vi "Experiment header-Save_Load STATS section.vi"(4 "Logging queue element":T2={"Imaging Protocol"=enum."Live Imaging", "Number of Trials"=0, "Frame Size"=0, "# Averaged frames"=0, "Dwell time (us)"=0.1, "Index of Z-plane"=0, "Timelapse?"=FALSE, "Logging process is active"=FALSE, "Speed logging enabled"=FALSE, "tdms file ref"=refnum, "path"=path "", "Trial Number"=0, "Expected # points acquired"=FALSE, "Manually stopped"=FALSE, "Ch0 data"=[], "Ch1 data"=[], "Last trial"=FALSE, "Points acquired"={"Ch0 last trial"=0, "Ch1 last trial"=0, "All trials"=0}} {"Frame Size" items=["100X100"=100, "128X128"=128, "200X200"=200, "256X256"=256, "512X512"=512, "1024x1024"=1024, "2048x2048"=2048]; "Dwell time (us)" format="%#.6g"}, 8 "error in (no error)":errorcluster, 10 "Function":enum16{"Write", "Read"}(ring), 11 "Experiment folder path":path) -> (0 "error out":errorcluster, 1 "Read values":T1, 2 "Acquisition time unknown":bool)   [LabVIEW 2013]
uses:
  Typedefs/Logging queue element.ctl
  Typedefs/Imaging Protocols enum.ctl
  Typedefs/Frame Size.ctl
  Typedefs/Acquired points count.ctl
  Typedefs/Test header stats cluster.ctl
  <vilib>/Utility/config.llb/Read Key (Double).vi
  <vilib>/Utility/config.llb/Write Key (Double).vi
  Global Variables/General Globals.vi
  <vilib>/Utility/config.llb/NI_LVConfig.lvlib
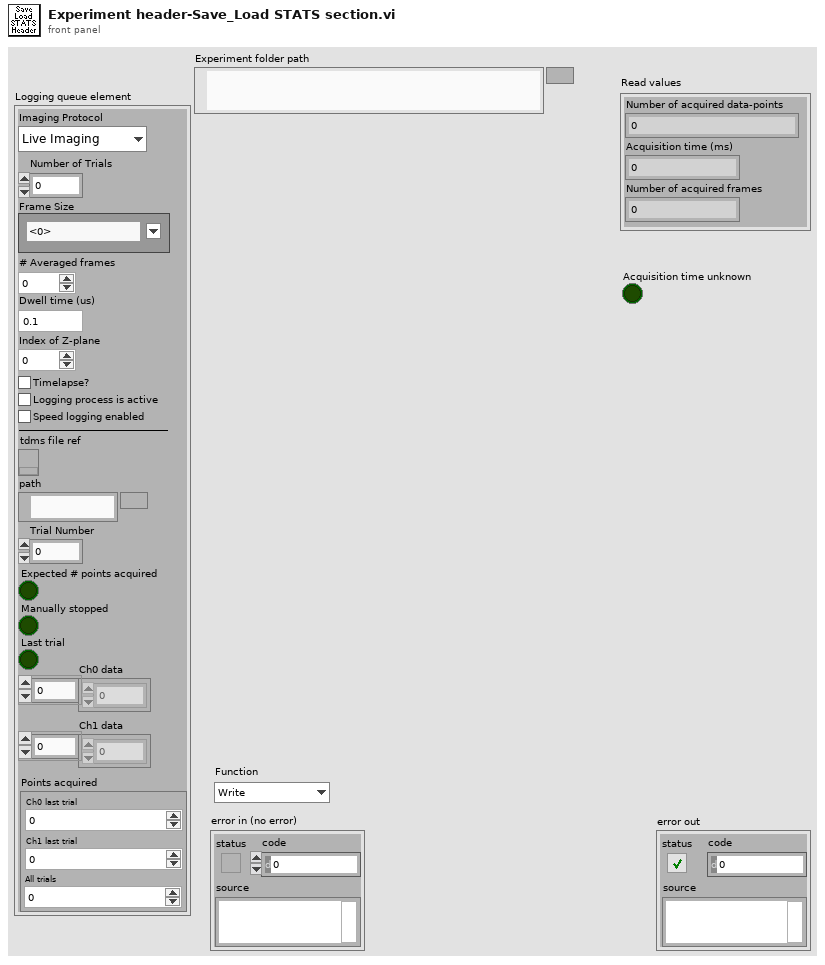
[diagram p1: front panel]
types:
  T1 = typedef "Test header stats cluster.ctl" = cluster{"Number of acquired data-points":dbl, "Acquisition time (ms)":dbl, "Number of acquired frames":dbl}
  T2 = typedef "Logging queue element.ctl" = cluster{"Imaging Protocol":T3, "Number of Trials":u16, "Frame Size":T4, "# Averaged frames":u16, "Dwell time (us)":dbl, "Index of Z-plane":i32, "Timelapse?":bool, "Logging process is active":bool, "Speed logging enabled":bool, "tdms file ref":refnum<k34>, "path":path, "Trial Number":i32, "Expected # points acquired":bool, "Manually stopped":bool, "Ch0 data":u32[], "Ch1 data":u32[], "Last trial":bool, "Points acquired":T5}
  T3 = typedef "Imaging Protocols enum.ctl" = enum16{"AOL Z-Stack", "Motor Z Stack", "Functional Acquisition", "Single Plane Acquisition", "Volume Acquisition", "Live Imaging", "Live Plane Imaging", "Live Volume Imaging"}
  T4 = typedef "Frame Size.ctl" = u16
  T5 = typedef "Acquired points count.ctl" = cluster{"Ch0 last trial":u64, "Ch1 last trial":u64, "All trials":u64}
  T6 = typedef "Fixed strings.ctl" = cluster{"ROI file name":string, "Normalised ROI file name":string, "Zplane Pockels values file name":string, "Functional data folder name":string, "Experiment Header file name":string, "Z-stack images folder name":string, "Groups setup rel. path":string, "Groups text file rel. path":string, "TDMS files folder name (F.img)":string, "TDMS files folder name (V.acq)":string, "TDMS files folder name (Pl.acq)":string, "Cycle rel times sequence file":string, "Dynamically called VIs folder name":string, "Time Series folder base name":string}
  T7 = typedef "NI_LVConfig.lvlib/Config Data RefNum.ctl" = refnum<k1>
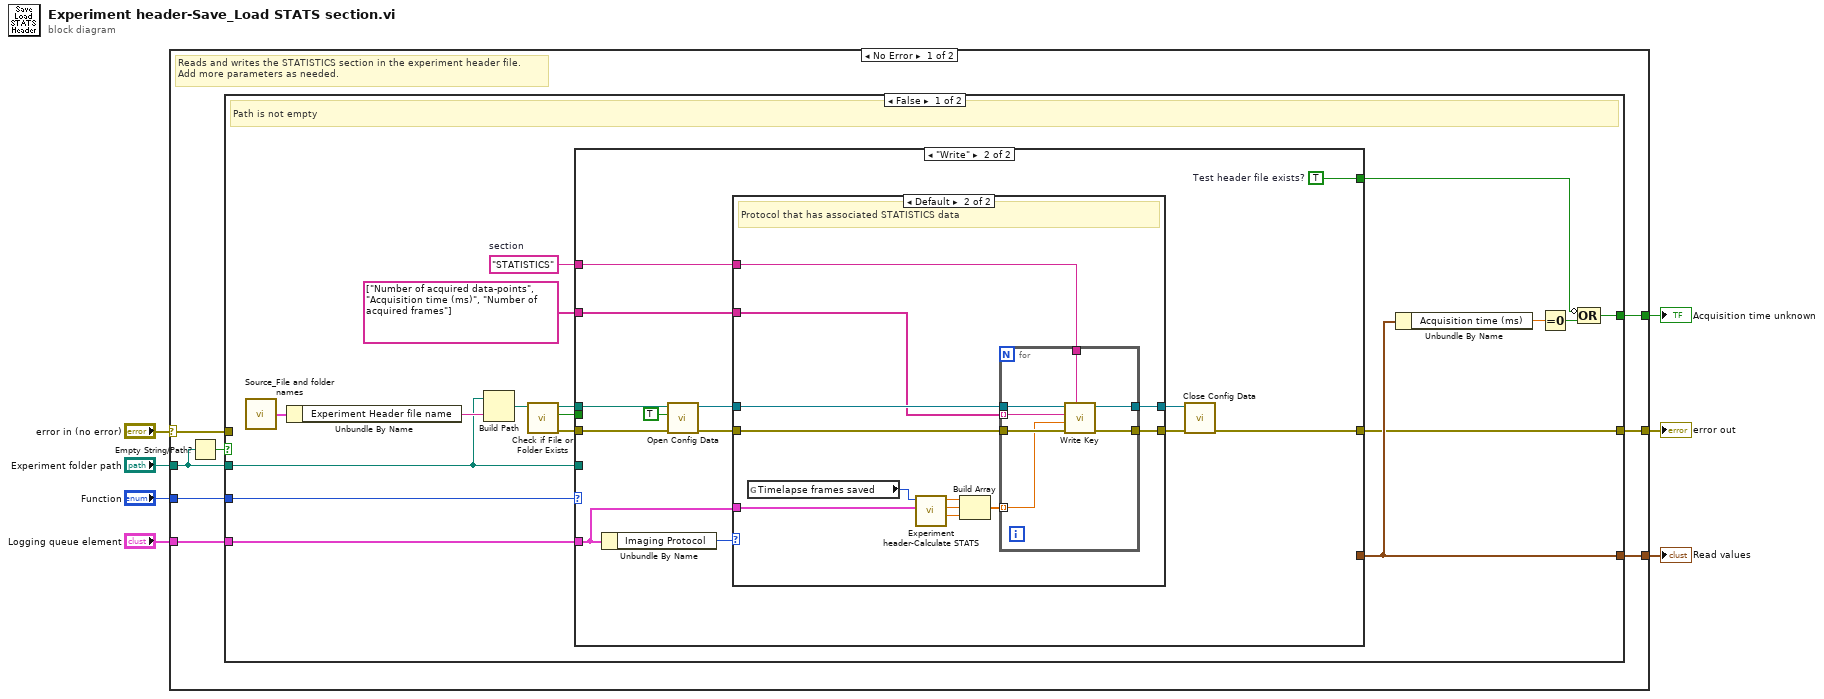
[diagram p0: block diagram]
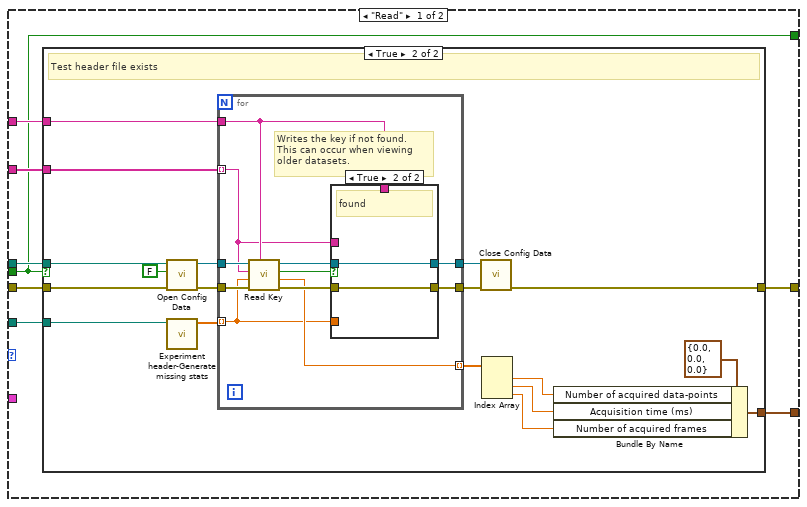
[diagram p2: hidden frame]
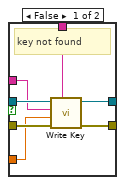
[diagram p4: hidden frame]
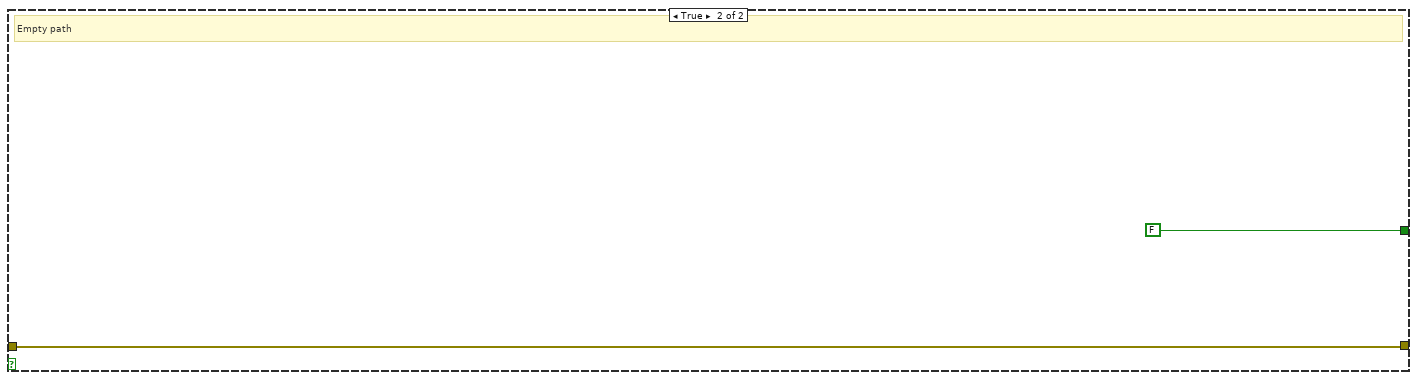
[diagram p6: hidden frame]
diagram:
  n1 = case shown="No Error" "error in (no error)" {
    selector: "error in (no error)" -> [w9 w116]
    tunnel: [w15 w116] -> w7
    tunnel: "Function" -> [w14 _]
    tunnel: "Experiment folder path" -> [w10 _]
    tunnel: "Logging queue element" -> [w13 _]
    tunnel: [w12 _] -> w3
    tunnel: [w8 _] -> w2
    frame No Error {
      # "Reads and writes the STATISTICS section in the experiment header file.\nAdd more parameters as needed."
      n2 = Empty String/Path?(string/path=w10) -> (empty?=w11:bool)
      n3 = case shown="False" w11 {
        tunnel: [w17 w115] -> w15
        tunnel: w14 -> [w21 _]
        tunnel: w10 -> [w22 _]
        tunnel: w13 -> [w23 _]
        tunnel: [w28 _] -> w12
        tunnel: w9 -> [_ w115]
        tunnel: [w25 FALSE ("File not found")] -> w8
        frame False {
          w24 = "STATISTICS"  # section
          # "Path is not empty"
          n4 = call "Source_File and folder names.vi"() -> ("Fixed strings"=w30:T6)  [unwired: 1 in]
          n5 = Unbundle By Name(w30) -> ("Experiment Header file name"=w31:string)
          n6 = Build Path(base path=w22, name or relative path=w31) -> (appended path=w29:path)
          n7 = call <vilib>:"Check if File or Folder Exists.vi"("path"=w29) -> ("error out"=w18:errorcluster, "file or folder exists?"=w20:bool, "dup path"=w19:path)  [unwired: 8 in]
          n8 = case shown="\"Write\"" w21 {
            tunnel: [w39 w81] -> w17
            tunnel: w18 -> [w40 w86]
            tunnel: w24 -> [w38 w92]
            tunnel: string[] ["Number of acquired data-points", "Acquisition time (ms)", "Number of acquired frames"] -> [w37 w91]
            tunnel: [w36 _] -> w28
            tunnel: w23 -> [_ w89]
            tunnel: w22 -> [w35 _]
            tunnel: w20 -> [w33 _]
            tunnel: w19 -> [w34 w87]
            tunnel: [w33 w83] -> w16
            frame "Read" {
              n9 = case shown="True" w33 {
                tunnel: w40 -> [w41 w46]
                tunnel: [w41 w42] -> w39
                tunnel: w38 -> [_ w59]
                tunnel: w37 -> [_ w58]
                tunnel: [_ w56] -> w36
                tunnel: w35 -> [_ w50]
                tunnel: w34 -> [_ w49]
                frame False {
                  # "Test header file doesnot exist"
                }
                frame True {
                  # "Test header file exists"
                  n10 = call <vilib>:"Open Config Data.vi"("error in (no error)"=w46, "create file if necessary (T)"=FALSE, "configuration file path"=w49) -> ("error out"=w45:errorcluster, "refnum"=w47:T7)  [unwired: 6 in, 1 out]
                  n11 = call "Experiment header-Generate missing stats.vi"("Experiment folder path"=w50) -> ("STATS array"=w51:dbl[])  [unwired: 10 in]
                  n12 = for {
                    tunnel: w47 -> [w70]
                    tunnel: w45 -> [w69]
                    tunnel: [w66] -> w44
                    tunnel: [w65] -> w43
                    tunnel: w59 -> [w64]
                    tunnel: [w62] -> w55 mode=indexing
                    tunnel: w51 -> [w60] mode=indexing
                    tunnel: w58 -> [w61] mode=indexing
                    # "Writes the key if not found.\nThis can occur when viewing older datasets."
                    n13 = call-poly <vilib>:"Read Key.vi"("section"=w64, "error in (no error)"=w69, "default value"=w60, "key"=w61, "refnum"=w70) -> ("error out"=w67:errorcluster, "value"=w62:dbl, "found?"=w63:bool, "refnum out"=w68:T7)  [unwired: 3 in]
                    n14 = case shown="True" w63 {
                      tunnel: w68 -> [w77 w79]
                      tunnel: w67 -> [w76 w78]
                      tunnel: [w75 w79] -> w66
                      tunnel: [w74 w78] -> w65
                      tunnel: w64 -> [w73 _]
                      tunnel: w61 -> [w72 _]
                      tunnel: w60 -> [w71 _]
                      frame False {
                        # "key not found"
                        n15 = call-poly <vilib>:"Write Key.vi"("section"=w73, "error in (no error)"=w76, "value"=w71, "key"=w72, "refnum"=w77) -> ("error out"=w74:errorcluster, "refnum out"=w75:T7)  [unwired: 4 in, 1 out]
                      }
                      frame True {
                        # "found"
                      }
                    }
                  }
                  n16 = call <vilib>:"Close Config Data.vi"("error in (no error)"=w43, "refnum"=w44) -> ("error out"=w42:errorcluster)  [unwired: 8 in, 1 out]
                  n17 = Index Array(array=w55) -> (element #1=w52:dbl, element #2=w54:dbl, element #3=w53:dbl)  [unwired: 3 in]
                  n18 = Bundle By Name(cluster=T1 {"Number of acquired data-points"=0.0, "Acquisition time (ms)"=0.0, "Number of acquired frames"=0.0} ("Read values"), "Number of acquired data-points"=w52, "Acquisition time (ms)"=w54, "Number of acquired frames"=w53) -> (w56:T1)
                }
              }
            }
            frame "Write" {
              w83 = TRUE  # Test header file exists?
              n19 = Unbundle By Name(w89) -> ("Imaging Protocol"=w90:T3)
              n20 = call <vilib>:"Open Config Data.vi"("error in (no error)"=w86, "create file if necessary (T)"=TRUE, "configuration file path"=w87) -> ("error out"=w85:errorcluster, "refnum"=w88:T7)  [unwired: 6 in, 1 out]
              n21 = case shown="Default" w90 {
                tunnel: w88 -> [w94 w106]
                tunnel: w85 -> [w93 w105]
                tunnel: w92 -> [_ w104]
                tunnel: [w93 w103] -> w80
                tunnel: [w94 w102] -> w82
                tunnel: w91 -> [_ w101]
                tunnel: w89 -> [_ w96]
                frame "AOL Z-Stack", "Motor Z Stack" {
                  # "Protocols without associated STATISTICS data"
                }
                frame Default {
                  # "Protocol that has associated STATISTICS data"
                  n22 = global read "General Globals.vi" "Timelapse frames saved"() -> (w95:u32)
                  n23 = call "Experiment header-Calculate STATS.vi"("Logging queue element"=w96, "Timelapse frames saved"=w95) -> ("Number of acquired frames"=w98:dbl, "Acquisition time (ms)"=w100:dbl, "Total number of points acquired (Ch0)"=w99:dbl)  [unwired: 7 in]
                  n24 = Build Array(w99, w100, w98) -> (w97:dbl[])
                  n25 = for {
                    tunnel: w106 -> [w113]
                    tunnel: w105 -> [w112]
                    tunnel: w101 -> [w111] mode=indexing
                    tunnel: w104 -> [w110]
                    tunnel: [w109] -> w103
                    tunnel: [w108] -> w102
                    tunnel: w97 -> [w107] mode=indexing
                    n26 = call-poly <vilib>:"Write Key.vi"("section"=w110, "error in (no error)"=w112, "value"=w107, "key"=w111, "refnum"=w113) -> ("error out"=w109:errorcluster, "refnum out"=w108:T7)  [unwired: 4 in, 1 out]
                  }
                }
              }
              n27 = call <vilib>:"Close Config Data.vi"("error in (no error)"=w80, "refnum"=w82) -> ("error out"=w81:errorcluster)  [unwired: 8 in, 1 out]
            }
          }
          n28 = Unbundle By Name(w28) -> ("Acquisition time (ms)"=w27:dbl)
          n29 = Equal To 0?(x=w27) -> (x = 0?=w26:bool)
          n30 = Compound Arithmetic op=OR(invert w16, w26) -> (w25:bool)
        }
        frame True {
          # "Empty path"
        }
      }
    }
    frame Error {
    }
  }
  "error out" <- w7
  "Read values" <- w3
  "Acquisition time unknown" <- w2
